vi "Test 3 Compare Different Types.vi"(8 "error in (no error)":errorcluster, 11 "Test Case In":refnum<class "Day 7 Test.lvclass">) -> (0 "error out":errorcluster, 3 "Test Case Out":refnum<class "Day 7 Test.lvclass">)   [LabVIEW 2020, in "Day 7 Test.lvclass"]
uses:
  Day 7 Test.lvclass
  C:/Program Files (x86)/National Instruments/LabVIEW 2020/vi.lib/Astemes/LUnit/Test Case.lvclass
  <vilib>/Astemes/LUnit/Test Case.lvclass/Test Case.ctl
  <vilib>/Astemes/LUnit/Append Fail Result.vi
  <vilib>/Astemes/LUnit/Append Pass Result.vi
  Day 7 Test.lvclass/Day 7 Test.ctl
  Hand/Hand.lvclass
  <vilib>/Astemes/LUnit/Test Case.lvclass
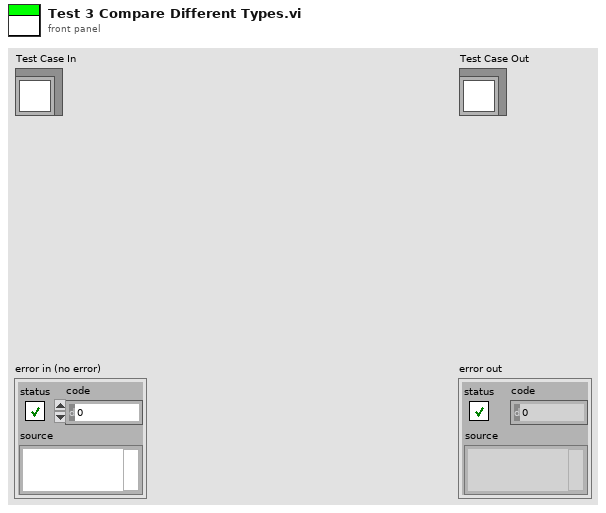
[diagram p1: front panel]
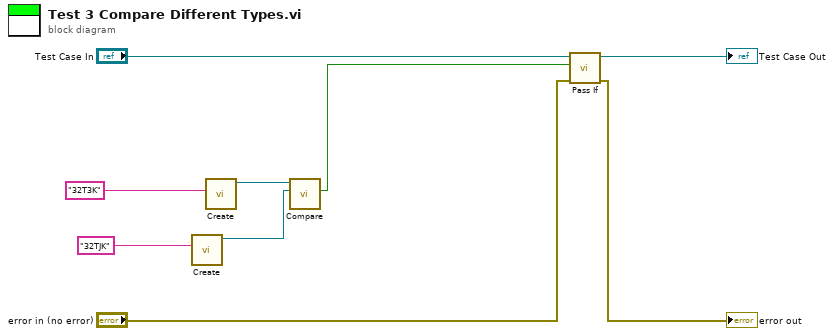
[diagram p0: block diagram]
diagram:
  n1 = call "Create.vi"("Input"="32TJK") -> ("Hand"=w2:refnum<class "Hand.lvclass">)  [unwired: 9 in, 1 out]
  n2 = call "Create.vi"("Input"="32T3K") -> ("Hand"=w3:refnum<class "Hand.lvclass">)  [unwired: 9 in, 1 out]
  n3 = call "Compare.vi"("Hand in 2"=w2, "Hand in"=w3) -> ("Higher?"=w1:bool)  [unwired: 7 in, 2 out]
  n4 = call <vilib>:"Pass If.vi"("error in (no error)"="error in (no error)", "Pass?"=w1, "LUnit Test Case In"="Test Case In") -> ("error out"=→"error out":errorcluster, "LUnit Test Case Out"=→"Test Case Out":refnum<class "Day 7 Test.lvclass">)  [unwired: 7 in]
